vi "pb_select_board.vi"(1 "error in (no error)":errorcluster, 2 "Board to Address":i32) -> (0 "error out":errorcluster)   [LabVIEW 2013, in "PulseBlaster.lvlib"]
uses:
  PulseBlaster.lvlib
  spinapi.dll
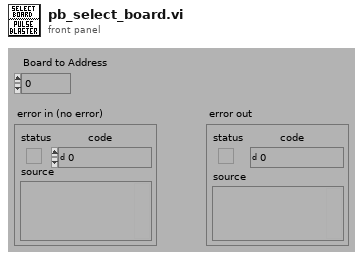
[diagram p1: front panel]
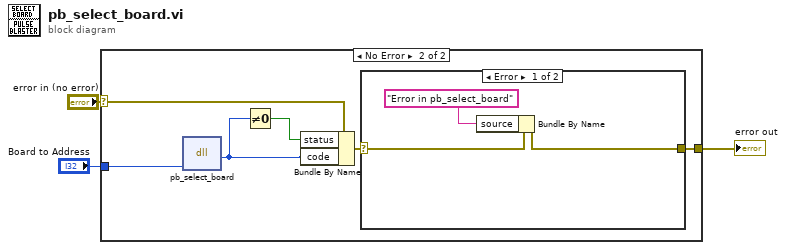
[diagram p0: block diagram]
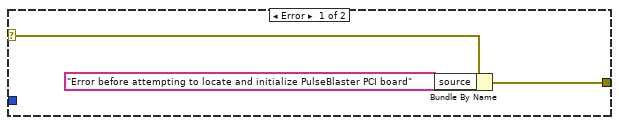
[diagram p2: hidden frame]
diagram:
  n1 = case shown="No Error" "error in (no error)" {
    selector: "error in (no error)" -> [w6 w12]
    tunnel: [w5 w9] -> w3
    tunnel: "Board to Address" -> [_ w7]
    frame Error {
      n2 = Bundle By Name(cluster=w6, "source"="Error before attempting to locate and initialize PulseBlaster PCI board") -> (w5:errorcluster)
    }
    frame No Error {
      n3 = dll-call lib="C:/Users/cherold/Documents/SVNrepo_local/branches/TableTest_Auto/codes/DeviceVIs/Pulseblaster/spinapi.dll" fn="pb_select_board"("board_num"=w7) -> ("return type"=w8:i32)  [unwired: 4 in, 2 out]
      n4 = Not Equal To 0?(x=w8) -> (x != 0?=w11:bool)
      n5 = Bundle By Name(cluster=w12, "status"=w11, "code"=w8) -> (w10:errorcluster)
      n6 = case shown="Error" w10 {
        selector: w10 -> [w15 w16]
        tunnel: [w13 w16] -> w9
        frame Error {
          n7 = Bundle By Name(cluster=w15, "source"="Error in pb_select_board") -> (w13:errorcluster)
        }
        frame No Error {
        }
      }
    }
  }
  "error out" <- w3
